vi "disp_var_unit.vi"() -> ()   [LabVIEW 2020]
panel:
  in  "Desired Variable":i32(listbox)
  out "Selected Fluid":string
  in  "Fluids List":i32(listbox)
  out "String":string
  in  "var_value":dbl format="%#_13g"
  out "Result":dbl
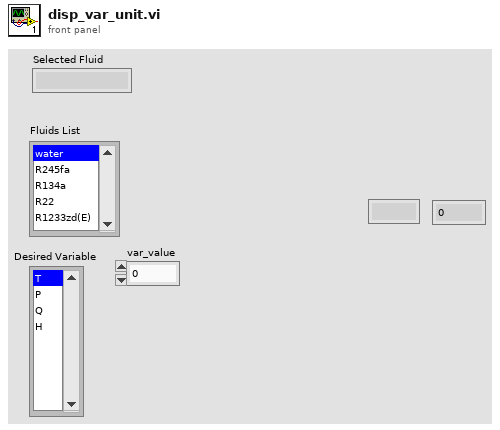
[diagram p1: front panel]
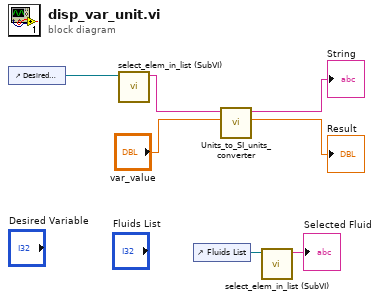
[diagram p0: block diagram]
diagram:
  n1 = control-ref of="Desired Variable"() -> (w2:refnum<vi>)
  n2 = call "select_elem_in_list (SubVI).vi"("ListBox in"=w2) -> ("String"=w1:string)  [unwired: 10 in]
  n3 = control-ref of="Fluids List"() -> (w4:refnum<vi>)
  n4 = call "Units_to_SI_units_converter.vi"("var_value in"="var_value", "String in"=w1) -> ("var_value out"=→"Result":dbl, "String out"=→"String":string)  [unwired: 8 in]
  n5 = call "select_elem_in_list (SubVI).vi"("ListBox in"=w4) -> ("String"=→"Selected Fluid":string)  [unwired: 10 in]
